vi "CreateEncoder.vi"(0 "Digital Module (Module 1)":T2, 1 "External Reset":T1={"DevStatus"={"status"=FALSE, "code"=0, "source"=""}, "AnalogTriggerMode?"=FALSE, "DigitalMode"={"Digital Module"=enum."Digital Module 1", "DIO Channel"=enum."Disabled"}, "AnalogTriggerMode"={"AnalogTriggerIndex"=enum."Trig 0", "OutputType"=enum."InWindow"}}, 2 "External Reset Active High":bool=TRUE, 3 "Minimum Rate":dbl=20.0, 5 "DIO A Channel":T10, 7 "DIO B Channel":T10, 9 "Invert Direction (False)":bool, 11 "error in (no error)":errorcluster, 12 "Decoding Type":T9=enum."4x", 13 "DistancePerCount":dbl=1.0, 14 "Number Samples to Average":u8=1 min=1 max=128) -> (4 "EncoderDevRef":T6={"DevStatus"={"status"=FALSE, "code"=0, "source"=""}, "EncoderIndex"=enum."Invalid", "CounterIndex"=enum."Invalid", "DistancePerCount"=1.0, "Decoding Type"=enum."4x"}, 15 "error out":errorcluster)   [LabVIEW 2013]
uses:
  <vilib>/Rock Robotics/SystemInterfaces/Typedef/FPGA_TypedefDigitalModule.ctl
  <vilib>/Rock Robotics/SystemInterfaces/DIO/FPGA_DIOChannel.ctl
  <vilib>/Rock Robotics/WPI/Encoder/WPI_EncoderType.ctl
  <vilib>/Rock Robotics/WPI/Encoder/WPI_EncoderDevRef.ctl
  <vilib>/Rock Robotics/SystemInterfaces/Encoder/FPGA_EncoderIdx.ctl
  <vilib>/Rock Robotics/SystemInterfaces/Counter/FPGA_CounterCtrSystemIndex.ctl
  <vilib>/Rock Robotics/SystemInterfaces/CounterEncoderSourceConvertion/FPGA_CounterEncoderSourceConvertionLVSourceType.ctl
  <vilib>/Rock Robotics/SystemInterfaces/DIO/FPGA_DIODigitalSourceChannel.ctl
  <vilib>/Rock Robotics/SystemInterfaces/AnalogTrigger/FPGA_AnalogTriggerIndex.ctl
  <vilib>/Rock Robotics/SystemInterfaces/AnalogTrigger/FPGA_AnalogTriggerOutType.ctl
  <vilib>/Rock Robotics/WPI/Counter/WPI_CounterDigitalInputToDigitalSource.vi
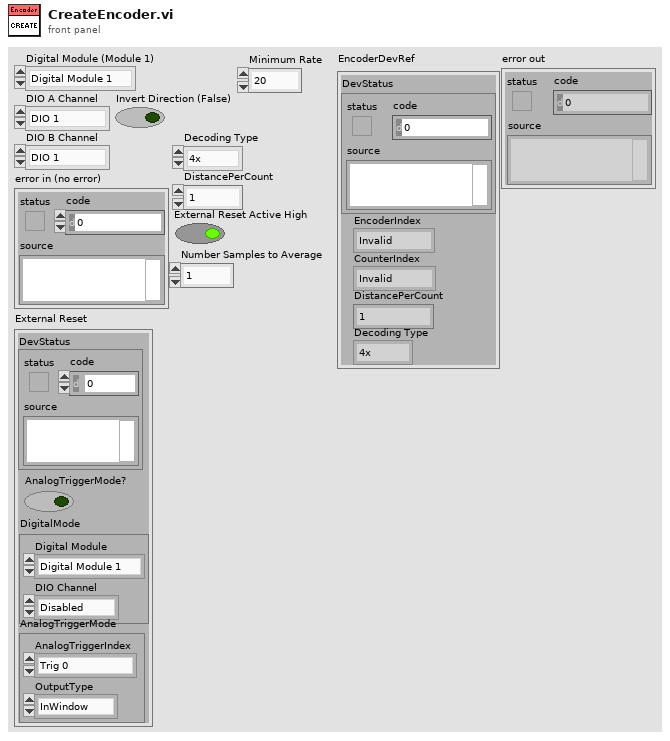
[diagram p1: front panel]
types:
  T1 = typedef "FPGA_CounterEncoderSourceConvertionLVSourceType.ctl" = cluster{"DevStatus":errorcluster, "AnalogTriggerMode?":bool, "DigitalMode":cluster{"Digital Module":T2, "DIO Channel":T3}, "AnalogTriggerMode":cluster{"AnalogTriggerIndex":T4, "OutputType":T5}}
  T2 = typedef "FPGA_TypedefDigitalModule.ctl" = enum16{"Digital Module 1", "Digital Module 2"}
  T3 = typedef "FPGA_DIODigitalSourceChannel.ctl" = enum8{"DIO 1", "DIO 2", "DIO 3", "DIO 4", "DIO 5", "DIO 6", "DIO 7", "DIO 8", "DIO 9", "DIO 10", "DIO 11", "DIO 12", "DIO 13", "DIO 14", "Disabled"}
  T4 = typedef "FPGA_AnalogTriggerIndex.ctl" = enum8{"Trig 0", "Trig 1", "Trig 2", "Trig 3", "Trig 4", "Trig 5", "Trig 6", "Trig 7", "Invalid"}
  T5 = typedef "FPGA_AnalogTriggerOutType.ctl" = enum16{"InWindow", "TriggerState", "Rising", "Falling"}
  T6 = typedef "WPI_EncoderDevRef.ctl" = cluster{"DevStatus":errorcluster, "EncoderIndex":T7, "CounterIndex":T8, "DistancePerCount":dbl, "Decoding Type":T9}
  T7 = typedef "FPGA_EncoderIdx.ctl" = enum8{"Enc 0", "Enc 1", "Enc 2", "Enc 3", "Invalid"}
  T8 = typedef "FPGA_CounterCtrSystemIndex.ctl" = enum8{"Ctr 0", "Ctr 1", "Ctr 2", "Ctr 3", "Ctr 4", "Ctr 5", "Ctr 6", "Ctr 7", "Invalid"}
  T9 = typedef "WPI_EncoderType.ctl" = enum16{"1x", "2x", "4x"}
  T10 = typedef "FPGA_DIOChannel.ctl" = enum8{"DIO 1", "DIO 2", "DIO 3", "DIO 4", "DIO 5", "DIO 6", "DIO 7", "DIO 8", "DIO 9", "DIO 10", "DIO 11", "DIO 12", "DIO 13", "DIO 14", "Invalid"}
  T11 = typedef "WPI_DigitalInputDevRef.ctl" = cluster{"DevStatus":errorcluster, "DIO Channel":T10, "Digital Module":T2}
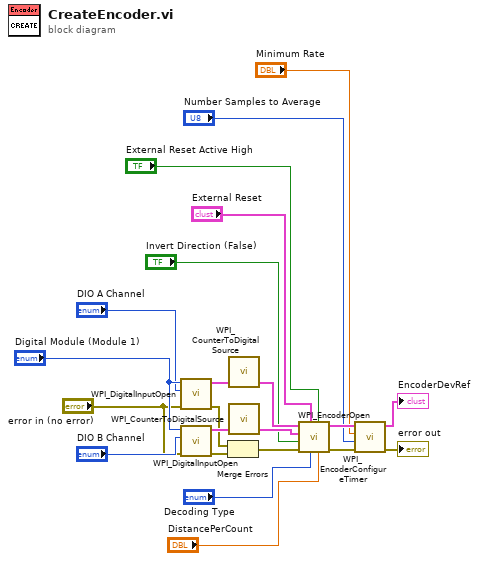
[diagram p0: block diagram]
diagram:
  n1 = call <vilib>:"WPI_DigitalInputOpen.vi"("error in (no error)"="error in (no error)", "DIO Channel"="DIO A Channel", "Digital Module (Module 1)"="Digital Module (Module 1)") -> ("error out"=w13:errorcluster, "DigitalInputDevRef"=w17:T11)  [unwired: 7 in]
  n2 = call <vilib>:"WPI_DigitalInputOpen.vi"("error in (no error)"="error in (no error)", "DIO Channel"="DIO B Channel", "Digital Module (Module 1)"="Digital Module (Module 1)") -> ("error out"=w12:errorcluster, "DigitalInputDevRef"=w18:T11)  [unwired: 7 in]
  n3 = Merge Errors(w13, w12) -> (w14:errorcluster)
  n4 = call-poly <vilib>:"WPI_CounterToDigitalSource.vi"("DigitalInputDevRef"=w17) -> ("Digital Source"=w16:T1)  [unwired: 6 in]
  n5 = call-poly <vilib>:"WPI_CounterToDigitalSource.vi"("DigitalInputDevRef"=w18) -> ("Digital Source"=w15:T1)  [unwired: 6 in]
  n6 = call <vilib>:"WPI_EncoderOpen.vi"("DistancePerCount"="DistancePerCount", "External Reset Active High"="External Reset Active High", "Decoding Type"="Decoding Type", "External Reset"="External Reset", "error in (no error)"=w14, "Invert Direction (False)"="Invert Direction (False)", "BSource"=w15, "ASource"=w16) -> ("error out"=w3:errorcluster, "EncoderDevRef"=w6:T6)  [unwired: 2 in]
  n7 = call <vilib>:"WPI_EncoderConfigureTimer.vi"("error in (no error)"=w3, "Number Samples to Average"="Number Samples to Average", "Minimum Rate"="Minimum Rate", "EncoderDevRef"=w6) -> ("error out"=→"error out":errorcluster, "EncoderDevRef"=→"EncoderDevRef":T6)  [unwired: 6 in]
